vi "Get Object from String.vi"(8 "error in":errorcluster, 9 "Sub-Index":string, 10 "Index":string, 11 "reference in":refnum<class "Electronic Datasheet.lvclass">) -> (0 "error out":errorcluster, 1 "OD Entry":refnum<class "OD Entry.lvclass">, 2 "Found?":bool, 3 "reference out":refnum<class "Electronic Datasheet.lvclass">)   [LabVIEW 2019, in "Electronic Datasheet.lvlib" / "Electronic Datasheet.lvclass"]
doc: "Get object from dictionary from strings in hex format"
uses:
  Electronic Datasheet.lvclass
  Core/OD Entry/OD Entry.lvclass
  Core/Sorted Object Dictionary/Sorted Object Dictionary.lvclass
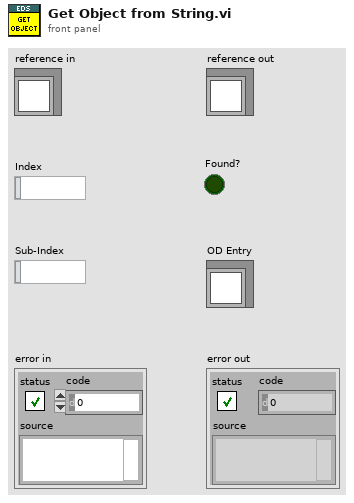
[diagram p1: front panel]
types:
  T1 = typedef "Electronic Datasheet.lvlib/Electronic Datasheet.lvclass/ObjectAttributes.ctl" = cluster{"EDS File Path":path, "Object Dict":refnum<class "Dictionary.lvclass">, "Sorted Object Dict":refnum<class "Sorted Object Dictionary.lvclass">, "Device Info":refnum<class "Device Info.lvclass">, "File Info":refnum<class "File Info.lvclass">}
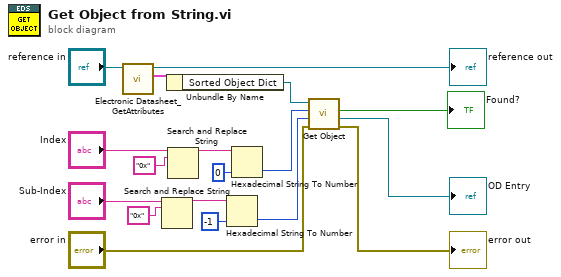
[diagram p0: block diagram]
diagram:
  n1 = call "Electronic Datasheet_GetAttributes.vi"("reference in"="reference in") -> ("Data"=w2:T1, "reference out"=→"reference out":refnum<class "Electronic Datasheet.lvclass">)  [unwired: 7 in, 2 out]
  n2 = Search and Replace String(input string="Sub-Index", search string="0x" ("string")) -> (result string=w10:string)  [unwired: 6 in, 3 out]
  n3 = Unbundle By Name(w2) -> ("Sorted Object Dict"=w1:refnum<class "Sorted Object Dictionary.lvclass">)
  n4 = Search and Replace String(input string="Index", search string="0x" ("string")) -> (result string=w15:string)  [unwired: 6 in, 3 out]
  n5 = Hexadecimal String To Number(string=w10, default (0uL)=i16 -1) -> (number=w9:i16)  [unwired: 1 in, 1 out]
  n6 = Hexadecimal String To Number(string=w15, default (0uL)=u16 0) -> (number=w14:u16)  [unwired: 1 in, 1 out]
  n7 = call "Get Object.vi"("error in"="error in", "Sub-Index"=w9, "Index"=w14, "Sorted Object Dictionary in"=w1) -> ("error out"=→"error out":errorcluster, "OD Entry"=→"OD Entry":refnum<class "OD Entry.lvclass">, "Found?"=→"Found?":bool)  [unwired: 4 in, 1 out]
